vi "DSE7_CS.vi"(8 "error in (no error)":errorcluster caption="err in", 10 "Weibull (paramètres)":T1) -> (0 "error out":errorcluster caption="err out", 2 "sigma":dbl, 3 "MTTF":dbl)   [LabVIEW 2010, in "lv_02.lvlib"]
doc: "Ce VI calcule l'espérance mathématique et la variance du modèle de Weibull à partir des paramètres (p_Lw)"
uses:
  p_5E7_LW.ctl
  lv_02.lvlib
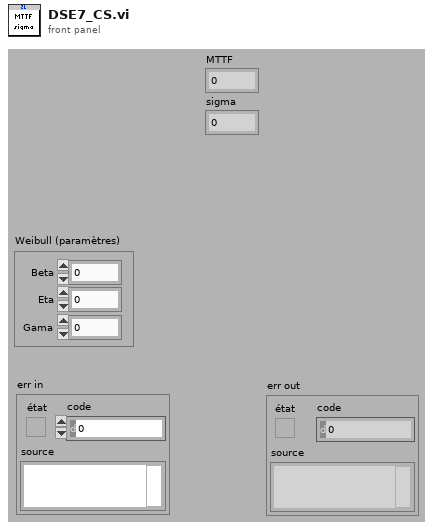
[diagram p1: front panel]
types:
  T1 = typedef "lv_02.lvlib/p_5E7_LW.ctl" = cluster{"Beta":dbl, "Eta":dbl, "Gama":dbl}
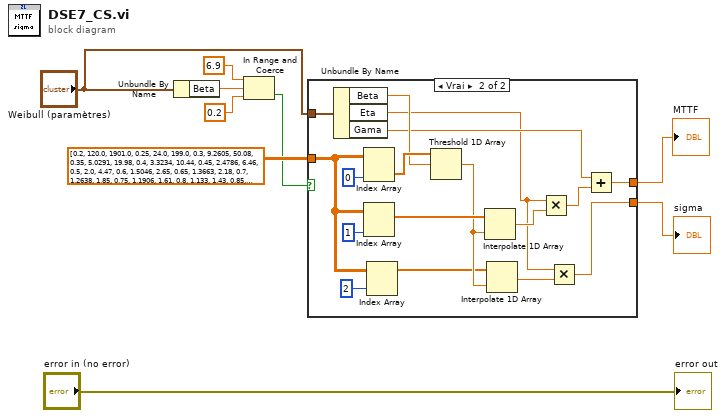
[diagram p0: block diagram]
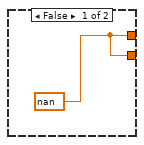
[diagram p2: hidden frame]
diagram:
  n1 = Unbundle By Name("Weibull (paramètres)") -> ("Beta"=w8:dbl)
  n2 = In Range and Coerce(upper limit=6.9 ("limite supérieure"), x=w8, lower limit=0.2 ("limite supérieure")) -> (In Range?=w5:bool)  [unwired: 1 out]
  n3 = case shown="Vrai" w5 {
    tunnel: dbl[][] [[0.2, 120.0, 1901.0], [0.25, 24.0, 199.0], [0.3, 9.2605, 50.08], [0.35, 5.0291, 19.98], [0.4, 3.3234, 10.44], [0.45, 2.4786, 6.46], [0.5, 2.0, 4.47], [0.6, 1.5046, 2.65], [0.65, 1.3663, 2.18], [0.7, 1.2638, 1.85], [0.75, 1.1906, 1.61], [0.8, 1.133, 1.43], [0.85, 1.088, 1.29], [0.9, 1.0522, 1.17], [0.95, 1.0234, 1.08], [1.0, 1.0, 1.0], [1.05, 0.9603, 0.934], [1.1, 0.9649, 0.878], [1.15, 0.9517, 0.83], [1.2, 0.9407, 0.787], [1.25, 0.9314, 0.75], [1.3, 0.9236, 0.716], [1.35, 0.917, 0.687], [1.4, 0.9114, 0.66], [1.45, 0.9067, 0.635], [1.5, 0.9027, 0.613], [1.55, 0.8994, 0.593], [1.6, 0.8966, 0.574], [1.65, 0.8942, 0.556], [1.7, 0.8922, 0.54], [1.75, 0.8906, 0.525], [1.8, 0.8893, 0.511], [1.85, 0.8882, 0.498], [1.9, 0.8874, 0.486], [1.95, 0.8867, 0.474], [2.0, 0.8862, 0.463], [2.1, 0.8857, 0.443], [2.2, 0.8856, 0.425], [2.3, 0.8859, 0.409], [2.4, 0.8865, 0.393], [2.5, 0.8873, 0.38], [2.6, 0.8882, 0.367], [2.7, 0.8893, 0.355], [2.8, 0.8905, 0.344], [2.9, 0.8917, 0.334], [3.0, 0.893, 0.325], [3.1, 0.8943, 0.316], [3.2, 0.8957, 0.307], [3.3, 0.897, 0.299], [3.4, 0.8984, 0.292], [3.5, 0.8997, 0.285], [3.6, 0.9011, 0.278], [3.7, 0.9025, 0.272], [3.8, 0.9038, 0.266], [3.9, 0.9051, 0.26], [4.0, 0.9064, 0.254], [4.2, 0.9089, 0.244], [4.4, 0.9114, 0.235], [4.6, 0.9137, 0.226], [4.8, 0.916, 0.218], [5.0, 0.9182, 0.21], [5.2, 0.9202, 0.203], [5.4, 0.9222, 0.194], [5.6, 0.9241, 0.191], [5.8, 0.926, 0.185], [6.0, 0.9277, 0.18], [6.2, 0.9294, 0.175], [6.4, 0.931, 0.17], [6.6, 0.9325, 0.166], [6.8, 0.934, 0.161], [6.9, 0.9347, 0.16]] ("all rows") -> [_ w22]
    tunnel: [w10 w15] -> w3
    tunnel: [w10 w12] -> w2
    tunnel: "Weibull (paramètres)" -> [_ w11]
    frame False {
      w10 = nan
    }
    frame True {
      n4 = Unbundle By Name(w11) -> ("Beta"=w19:dbl, "Eta"=w13:dbl, "Gama"=w16:dbl)
      n5 = Index Array(array=w22, index (col)=0 ("indice désactivé (col)")) -> (element=w26:dbl[])  [unwired: 1 in]
      n6 = Index Array(array=w22, index (col)=1 ("indice désactivé (col)")) -> (element=w24:dbl[])  [unwired: 1 in]
      n7 = Index Array(array=w22, index (col)=2 ("indice désactivé (col)")) -> (element=w20:dbl[])  [unwired: 1 in]
      n8 = Threshold 1D Array(2:w19, 3:w26) -> (0:w21:dbl)  [unwired: 1 in]
      n9 = Interpolate 1D Array(1:w21, 2:w24) -> (0:w18:dbl)
      n10 = Interpolate 1D Array(1:w21, 2:w20) -> (0:w14:dbl)
      n11 = Multiply(x=w13, y=w18) -> (x*y=w17:dbl)
      n12 = Multiply(x=w13, y=w14) -> (x*y=w12:dbl)
      n13 = Add(x=w16, y=w17) -> (x+y=w15:dbl)
    }
  }
  "MTTF" <- w3
  "sigma" <- w2
  "error out" <- "error in (no error)"
